vi "Get position.vi"(8 "error in (no error)":errorcluster, 11 "AlphaStep One in":refnum<class "AlphaStep One.lvclass">) -> (0 "error out":errorcluster, 2 "Position (rev)":dbl, 3 "AlphaStep One out":refnum<class "AlphaStep One.lvclass">)   [LabVIEW 2015, in "AlphaStep One.lvclass"]
uses:
  AlphaStep One.lvclass
  AlphaStep One.lvclass/AlphaStep One.ctl
  Serial Device/Serial Device.lvclass
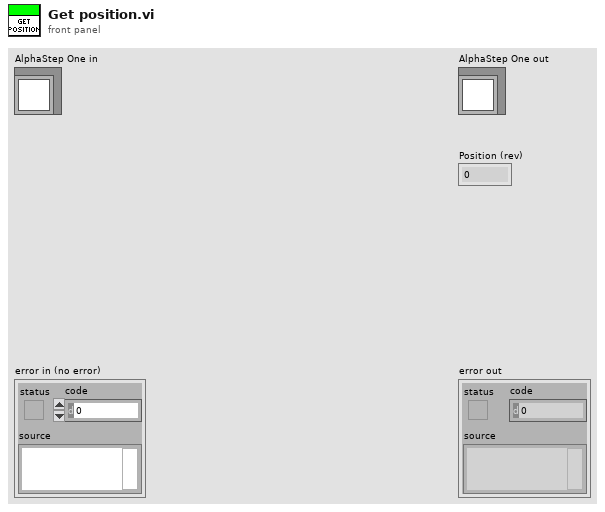
[diagram p1: front panel]
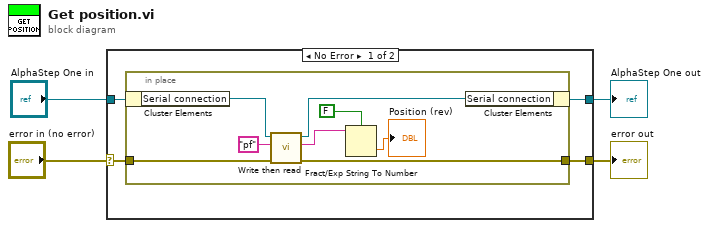
[diagram p0: block diagram]
diagram:
  n1 = case shown="No Error" "error in (no error)" {
    selector: "error in (no error)" -> [w7 w18]
    tunnel: [w6 w18] -> w3
    tunnel: [w5 w17] -> w1
    tunnel: "AlphaStep One in" -> [w8 w17]
    frame No Error {
      n2 = in-place {
        in-place-border: w7 -> [w15]
        in-place-border: [w14] -> w6
        n3 = in-place-cluster #1(w8) -> ("Serial connection"=w16:refnum<class "Serial Device.lvclass">)
        n4 = call "Write then read.vi"("error in (no error)"=w15, "TX Data"="pf", "Serial Device in"=w16) -> ("error out"=w14:errorcluster, "RX Data"=w12:string, "Serial Device out"=w10:refnum<class "Serial Device.lvclass">)  [unwired: 6 in]
        n5 = Fract/Exp String To Number(use system decimal point (T)=FALSE, string=w12) -> (number=→"Position (rev)":dbl)  [unwired: 2 in, 1 out]
        n6 = in-place-cluster #1("Serial connection"=w10) -> (w5:refnum<class "AlphaStep One.lvclass">)
      }
    }
    frame Error {
    }
  }
  "error out" <- w3
  "AlphaStep One out" <- w1
